vi "RMIO AI Convert.vi"(11 "AI [hexbits]":i16[](array[numeric])=[0, 0, 0, 0, 0, 0, 0, 0]) -> (3 "AI [V]":fxp<+/-,20,5>[](array[numeric]))   [LabVIEW 2015]
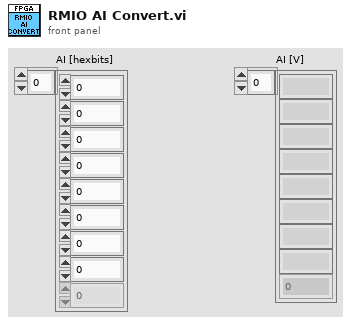
[diagram p1: front panel]
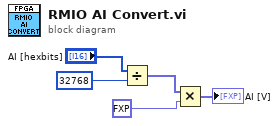
[diagram p0: block diagram]
diagram:
  n1 = Divide(x="AI [hexbits]", y=u32 32768) -> (x/y=w3:fxp<+/-,20,5>[])
  n2 = Multiply(x=w3, y=fxp<+/-,20,5> 10.0) -> (x*y=→"AI [V]":fxp<+/-,20,5>[])
